vi "Main.vi"() -> ()   [LabVIEW 2024]
uses:
  Pump Controls.ctl
  Pump Switch.ctl
  Pump Indicators.ctl
  Q Info.ctl
  App Data.ctl
  ffefbeac-5083-4d03-82bf-6186f2ceb5cf.vi
  e7fc6d58-ebef-41db-84b9-063138119824.vi
panel:
  in  "STOP":bool
  in  "Silence Alarm":bool
  out "Station Indicators":T1 {"Pump Water Level" scale=0.0..4.0}
  in  "Pump Controls":T2={"Lag Pump"=enum."OFF", "Lead Pump"=enum."OFF", "ALARM"=4.0, "LAG"=3.0, "LEAD"=2.0, "STOP"=1.0}
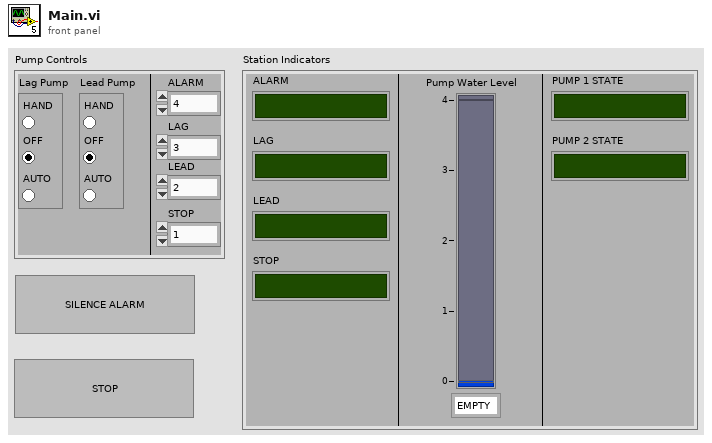
[diagram p1: front panel]
types:
  T1 = typedef "Pump Indicators.ctl" = cluster{"Pump Water Level":dbl, "ALARM":bool, "LAG":bool, "LEAD":bool, "STOP":bool, "PUMP 1 STATE":bool, "PUMP 2 STATE":bool}
  T2 = typedef "Pump Controls.ctl" = cluster{"Lag Pump":T3, "Lead Pump":T3, "ALARM":dbl, "LAG":dbl, "LEAD":dbl, "STOP":dbl}
  T3 = typedef "Pump Switch.ctl" = enum32{"HAND", "OFF", "AUTO"}
  T4 = typedef "App Data.ctl" = cluster{"Pump Station Controls":T2, "Pump Indicators":T1, "Alarm":refnum<notifier>, "Lag Start Time":timestamp, "Lead Start Time":timestamp, "Main Q":refnum<queue>}
  T5 = typedef "Q Info.ctl" = cluster{"State":string, "Data":variant}
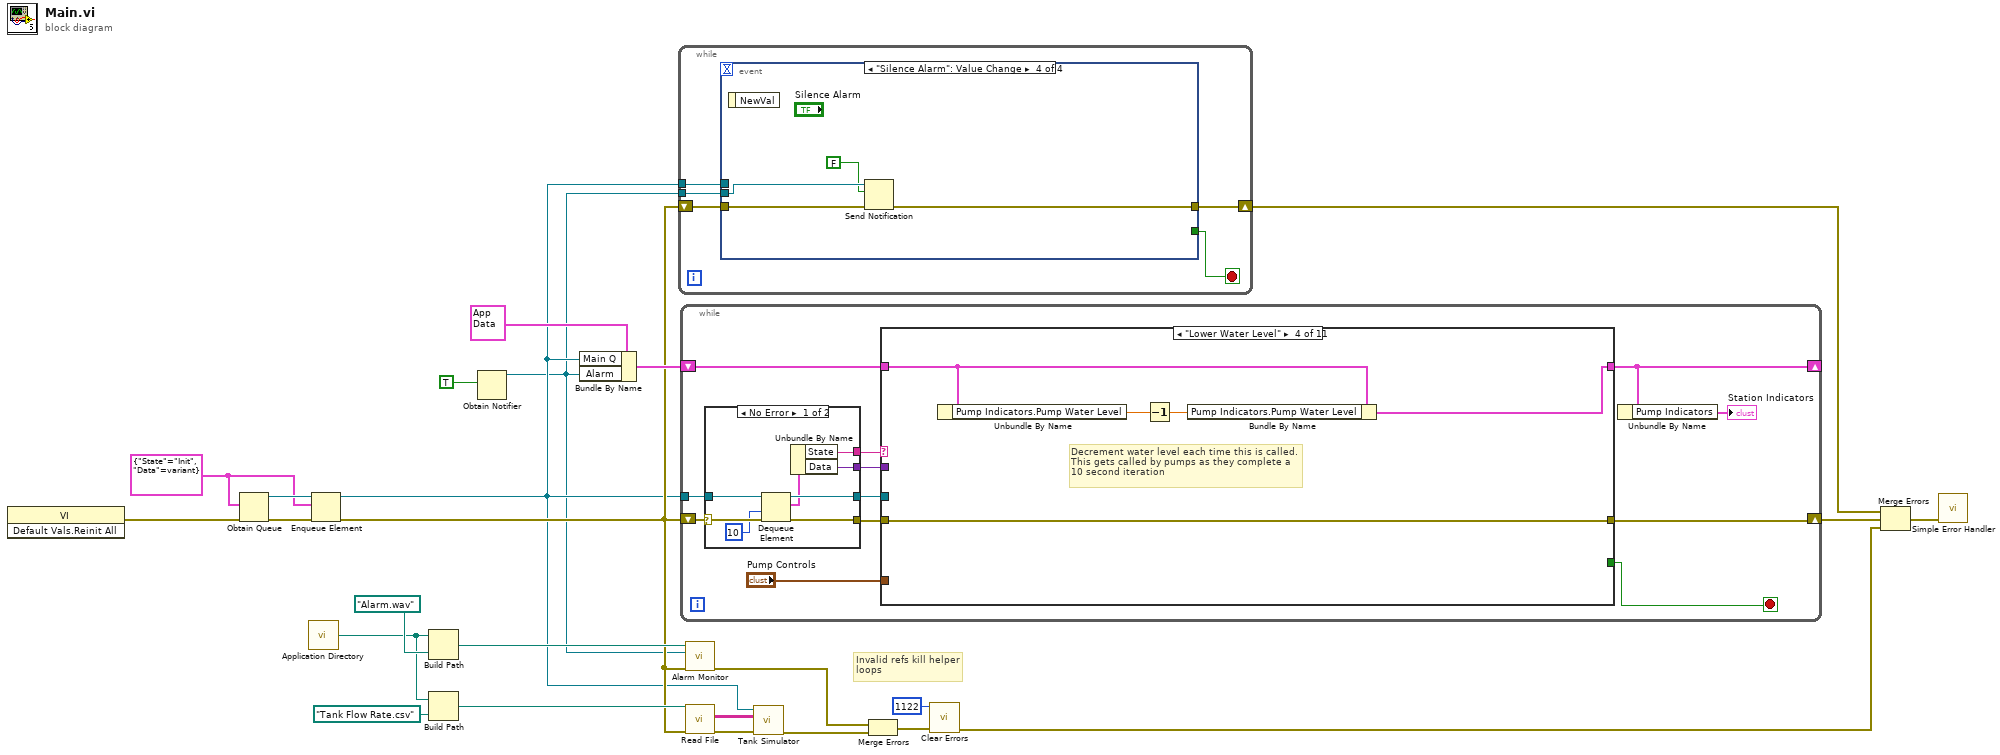
[diagram p0: block diagram]
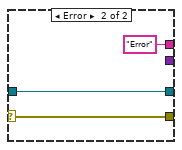
[diagram p2: hidden frame]
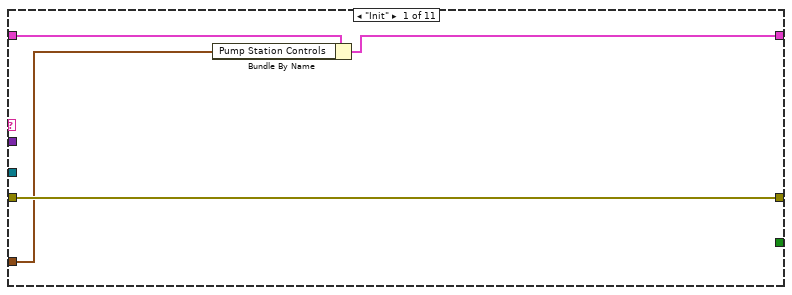
[diagram p3: hidden frame]
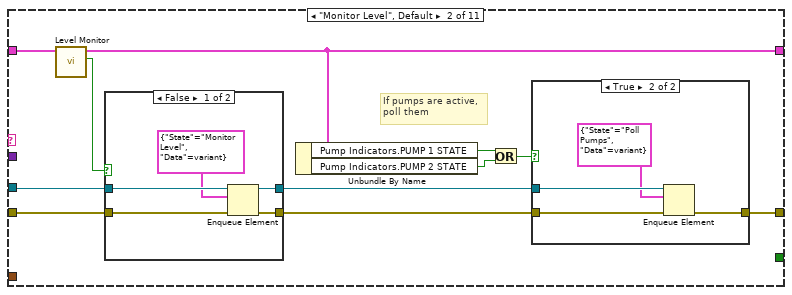
[diagram p4: hidden frame]
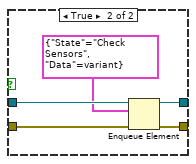
[diagram p6: hidden frame]
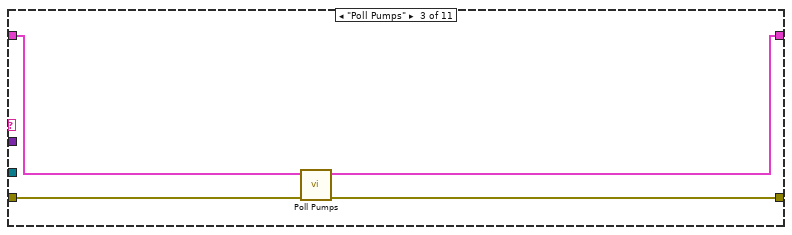
[diagram p7: hidden frame]
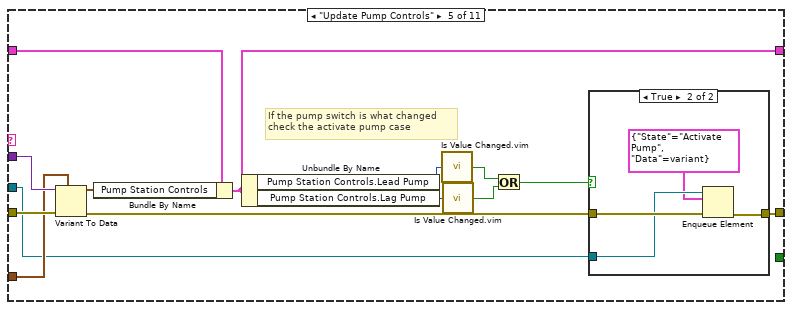
[diagram p8: hidden frame]
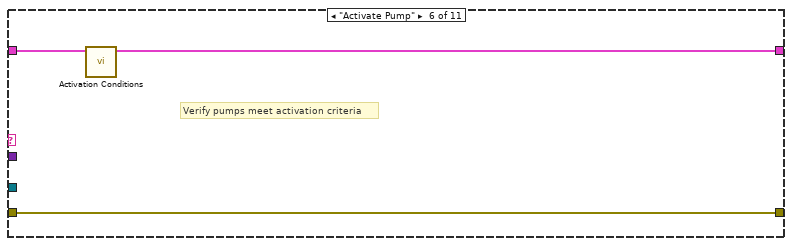
[diagram p10: hidden frame]
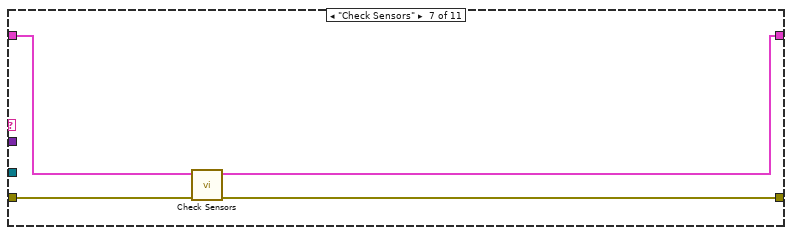
[diagram p11: hidden frame]
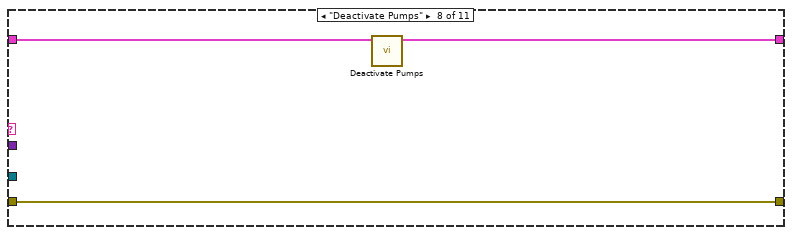
[diagram p12: hidden frame]
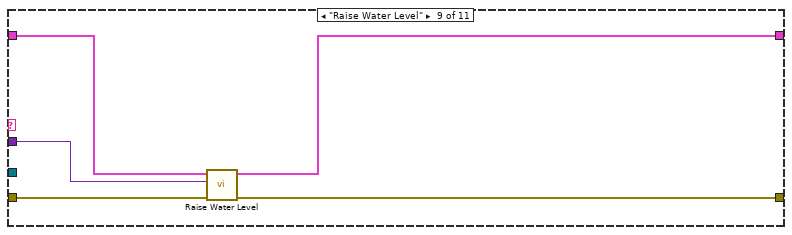
[diagram p13: hidden frame]
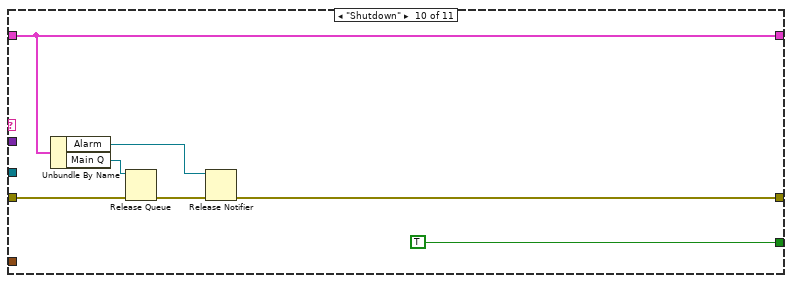
[diagram p14: hidden frame]
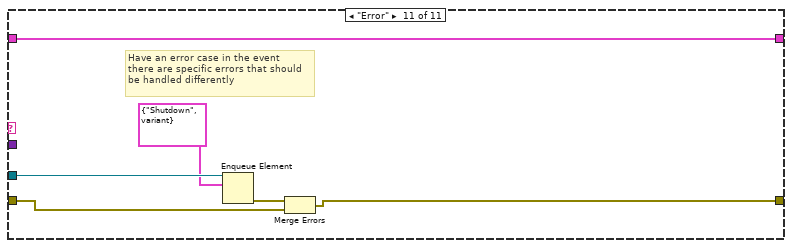
[diagram p15: hidden frame]
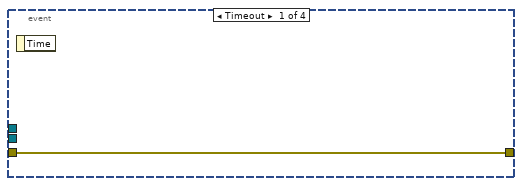
[diagram p16: hidden frame]
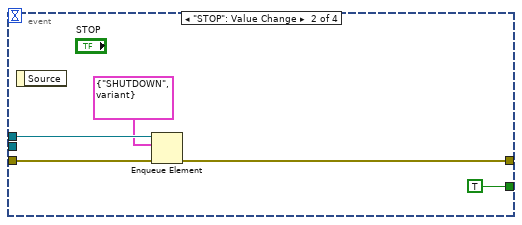
[diagram p17: hidden frame]
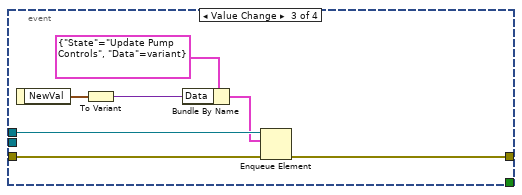
[diagram p18: hidden frame]
diagram:
  w23 = T5 {"State"="Init", "Data"=variant} ("Cluster")
  # "Invalid refs kill helper\nloops"
  n1 = invoke class="VI" method="Default Vals.Reinit All"() -> (error out=w2:errorcluster)  [unwired: 3 in, 2 out]
  n2 = Obtain Queue(element data type=w23, error in (no error)=w2) -> (queue out=w25:refnum<queue>, error out=w24:errorcluster)  [unwired: 3 in, 1 out]
  n3 = call <vilib>:"Application Directory.vi"() -> ("Application Directory"=w14:path)
  n4 = Enqueue Element(queue=w25, element=w23, error in (no error)=w24) -> (queue out=w8:refnum<queue>, error out=w11:errorcluster)  [unwired: 1 in, 1 out]
  n5 = Build Path(base path=w14, name or relative path=path "Alarm.wav") -> (appended path=w15:path)
  n6 = Build Path(base path=w14, name or relative path=path "Tank Flow Rate.csv") -> (appended path=w12:path)
  n7 = Obtain Notifier(notification data type=TRUE) -> (notifier out=w1:refnum<notifier>)  [unwired: 3 in, 2 out]
  n8 = Bundle By Name(cluster=T4 {"Pump Station Controls"={"Lag Pump"=enum."OFF", "Lead Pump"=enum."OFF", "ALARM"=0.0, "LAG"=0.0, "LEAD"=0.0, "STOP"=0.0}, "Pump Indicators"={"Pump Water Level"=0.0, "ALARM"=FALSE, "LAG"=FALSE, "LEAD"=FALSE, "STOP"=FALSE, "PUMP 1 STATE"=FALSE, "PUMP 2 STATE"=FALSE}, "Alarm"=refnum, "Lag Start Time"=timestamp(0 s since 1904-01-01), "Lead Start Time"=timestamp(0 s since 1904-01-01), "Main Q"=refnum} ("App Data"), "Main Q"=w8, "Alarm"=w1) -> (w18:T4)
  n9 = while {
    tunnel: w8 -> [w30]
    shift-right: [w27] -> w20
    shift-left: w11 -> [w29]
    tunnel: w1 -> [w26]
    stop <- w28 stop-if-true
    n10 = event shown="[3] \"Silence Alarm\": Value Change" {
      selector: _ -> [_ _ _ _]
      dyn-events: _ -> [_ _ _ _]
      timeout: _ -> [_ _ _ _]
      tunnel: w30 -> [_ w34 w42 _]
      tunnel: w29 -> [w31 w35 w43 w47]
      tunnel: [_ TRUE _ _] -> w28
      tunnel: [w31 w32 w37 w44] -> w27
      tunnel: w26 -> [_ _ _ w46]
      event Timeout {
        n11 = event-data() -> ()  [unwired: 1 in, 1 out]
      }
      event "STOP": Value Change {
        n12 = event-data() -> ()  [unwired: 1 in, 1 out]
        n13 = Enqueue Element(queue=w34, element=T5 {"State"="SHUTDOWN", "Data"=variant}, error in (no error)=w35) -> (error out=w32:errorcluster)  [unwired: 1 in, 2 out]
      }
      event Value Change {
        n14 = event-data() -> ("NewVal"=w40:T2)  [unwired: 1 in]
        n15 = To Variant(anything=w40) -> (Variant=w39:variant)
        n16 = Bundle By Name(cluster=T5 {"State"="Update Pump Controls", "Data"=variant} ("element"), "Data"=w39) -> (w38:T5)
        n17 = Enqueue Element(queue=w42, element=w38, error in (no error)=w43) -> (error out=w37:errorcluster)  [unwired: 1 in, 2 out]
      }
      event "Silence Alarm": Value Change {
        n18 = event-data() -> ()  [unwired: 1 in, 1 out]
        n19 = Send Notification(notification=FALSE, notifier=w46, error in (no error)=w47) -> (error out=w44:errorcluster)  [unwired: 1 out]
      }
    }
  }
  n20 = while {
    shift-right: [w54] -> w22
    shift-left: w11 -> [w59]
    tunnel: w8 -> [w58]
    shift-right: [w50] -> _
    shift-left: w18 -> [w52]
    stop <- w53 stop-if-true
    n21 = case shown="No Error" w59 {
      selector: w59 -> [w67 w70]
      tunnel: w58 -> [w66 w68]
      tunnel: [w65 w70] -> w56
      tunnel: [w64 w68] -> w57
      tunnel: [w62 "Error" ("State")] -> w55
      tunnel: [w61 _] -> w48
      frame No Error {
        n22 = Dequeue Element(queue=w66, timeout in ms (-1)=10, error in (no error)=w67) -> (queue out=w64:refnum<queue>, element=w63:T5, error out=w65:errorcluster)  [unwired: 1 out]
        n23 = Unbundle By Name(w63) -> ("State"=w62:string, "Data"=w61:variant)
      }
      frame Error {
      }
    }
    n24 = case shown="\"Lower Water Level\"" w55 {
      tunnel: w57 -> [_ w82 _ _ w113 _ _ _ _ _ w155]
      tunnel: w56 -> [w74 w84 w104 w105 w123 w129 w135 w136 w143 w149 w152]
      tunnel: [w74 w76 w103 w105 w114 w129 w134 w136 w139 w147 w156] -> w54
      tunnel: [_ _ _ _ _ _ _ _ _ TRUE _] -> w53
      tunnel: w52 -> [w73 w85 w102 w109 w112 w131 w133 w138 w142 w146 w151]
      tunnel: [w72 w81 w101 w108 w111 w130 w132 w137 w141 w146 w151] -> w50
      tunnel: "Pump Controls" -> [w71 _ _ _ w121 _ _ _ _ _ _]
      tunnel: w48 -> [_ _ _ _ w122 _ _ _ w140 _ _]
      frame "Init" {
        n25 = Bundle By Name(cluster=w73, "Pump Station Controls"=w71) -> (w72:T4)
      }
      frame "Monitor Level", Default {
        # "If pumps are active,\npoll them"
        n26 = call "Level Monitor.vi"("App Data"=w85) -> ("Sensor Change"=w83:bool, "App Data 2"=w81:T4)  [unwired: 9 in]
        n27 = case shown="False" w83 {
          tunnel: w84 -> [w95 w100]
          tunnel: w82 -> [w93 w99]
          tunnel: [w94 w98] -> w77
          tunnel: [w91 w96] -> w75
          frame False {
            n28 = Enqueue Element(queue=w93, element=T5 {"State"="Monitor Level", "Data"=variant}, error in (no error)=w95) -> (queue out=w91:refnum<queue>, error out=w94:errorcluster)  [unwired: 1 in, 1 out]
          }
          frame True {
            n29 = Enqueue Element(queue=w99, element=T5 {"State"="Check Sensors", "Data"=variant}, error in (no error)=w100) -> (queue out=w96:refnum<queue>, error out=w98:errorcluster)  [unwired: 1 in, 1 out]
          }
        }
        n30 = Unbundle By Name(w81) -> ("Pump Indicators.PUMP 1 STATE"=w79:bool, "Pump Indicators.PUMP 2 STATE"=w78:bool)
        n31 = Or(x=w79, y=w78) -> (x .or. y?=w80:bool)
        n32 = case shown="True" w80 {
          tunnel: w77 -> [w86 w90]
          tunnel: [w86 w89] -> w76
          tunnel: w75 -> [_ w88]
          frame False {
          }
          frame True {
            n33 = Enqueue Element(queue=w88, element=T5 {"State"="Poll Pumps", "Data"=variant}, error in (no error)=w90) -> (error out=w89:errorcluster)  [unwired: 1 in, 2 out]
          }
        }
      }
      frame "Poll Pumps" {
        n34 = call "Poll Pumps.vi"("error in (no error)"=w104, "App Data"=w102) -> ("error out"=w103:errorcluster, "App Data Out"=w101:T4)  [unwired: 8 in]
      }
      frame "Lower Water Level" {
        # "Decrement water level each time this is called.\nThis gets called by pumps as they complete a\n10 second iteration"
        n35 = Unbundle By Name(w109) -> ("Pump Indicators.Pump Water Level"=w107:dbl)
        n36 = Decrement(x=w107) -> (x-1=w106:dbl)
        n37 = Bundle By Name(cluster=w109, "Pump Indicators.Pump Water Level"=w106) -> (w108:T4)
      }
      frame "Update Pump Controls" {
        # "If the pump switch is what changed\ncheck the activate pump case"
        n38 = Variant To Data(error in=w123, type=w121, Variant=w122) -> (data=w120:T2, error out=w119:errorcluster)
        n39 = Bundle By Name(cluster=w112, "Pump Station Controls"=w120) -> (w111:T4)
        n40 = Unbundle By Name(w111) -> ("Pump Station Controls.Lead Pump"=w118:T3, "Pump Station Controls.Lag Pump"=w117:T3)
        n41 = call "Is Value Changed.vim"("value"=w118) -> ("changed or first call?"=w116:bool)
        n42 = call "Is Value Changed.vim"("value"=w117) -> ("changed or first call?"=w115:bool)
        n43 = Or(x=w116, y=w115) -> (x .or. y?=w110:bool)
        n44 = case shown="True" w110 {
          tunnel: w119 -> [w124 w128]
          tunnel: [w124 w127] -> w114
          tunnel: w113 -> [_ w126]
          frame False {
          }
          frame True {
            n45 = Enqueue Element(queue=w126, element=T5 {"State"="Activate Pump", "Data"=variant}, error in (no error)=w128) -> (error out=w127:errorcluster)  [unwired: 1 in, 2 out]
          }
        }
      }
      frame "Activate Pump" {
        # "Verify pumps meet activation criteria"
        n46 = call "Activation Conditions.vi"("App Data"=w131) -> ("App Data 2"=w130:T4)  [unwired: 10 in]
      }
      frame "Check Sensors" {
        n47 = call "Check Sensors.vi"("error in (no error)"=w135, "App Data in"=w133) -> ("error out"=w134:errorcluster, "App Data in 2"=w132:T4)  [unwired: 8 in]
      }
      frame "Deactivate Pumps" {
        n48 = call "Deactivate Pumps.vi"("App Data"=w138) -> ("App Data 2"=w137:T4)  [unwired: 10 in]
      }
      frame "Raise Water Level" {
        n49 = call "Raise Water Level.vi"("error in (no error)"=w143, "Data"=w140, "App Data"=w142) -> ("error out"=w139:errorcluster, "App Data 2"=w141:T4)  [unwired: 7 in]
      }
      frame "Shutdown" {
        n50 = Unbundle By Name(w146) -> ("Alarm"=w145:refnum<notifier>, "Main Q"=w144:refnum<queue>)
        n51 = Release Queue(queue=w144, error in (no error)=w149) -> (error out=w148:errorcluster)  [unwired: 1 in, 2 out]
        n52 = Release Notifier(notifier=w145, error in (no error)=w148) -> (error out=w147:errorcluster)  [unwired: 1 in, 2 out]
      }
      frame "Error" {
        # "Have an error case in the event\nthere are specific errors that should\nbe handled differently"
        n53 = Enqueue Element(queue=w155, element=T5 {"State"="Shutdown", "Data"=variant}) -> (error out=w153:errorcluster)  [unwired: 2 in, 2 out]
        n54 = Merge Errors(w153, w152) -> (w156:errorcluster)
      }
    }
    n55 = Unbundle By Name(w50) -> ("Pump Indicators"=→"Station Indicators":T1)
  }
  n56 = call "Alarm Monitor.vi"("error in (no error)"=w11, "Alarm"=w1, "Sound file"=w15) -> ("error out"=w6:errorcluster)  [unwired: 8 in]
  n57 = call "Read File.vi"("error in (no error)"=w11, "CSV File"=w12) -> ("error in (no error) 2"=w9:errorcluster, "Data"=w10:string[][])  [unwired: 8 in]
  n58 = call "Tank Simulator.vi"("error in (no error)"=w9, "Flow Rate Data"=w10, "queue out"=w8) -> ("error in (no error) 2"=w7:errorcluster)  [unwired: 8 in]
  n59 = Merge Errors(w6, w7) -> (w5:errorcluster)
  n60 = call <vilib>:"Clear Errors.vi"("error in (no error)"=w5, "specific error code to clear (0: all)"=1122) -> ("error out"=w3:errorcluster)  [unwired: 4 in, 1 out]
  n61 = Merge Errors(w20, w22, w3) -> (w21:errorcluster)
  n62 = call <vilib>:"Simple Error Handler.vi"("error in (no error)"=w21) -> ()  [unwired: 4 in, 5 out]
